vi "Cycle.vi"(8 "error in (no error)":errorcluster, 11 "BehaviorClassification In":refnum<class "BehaviorClassification.lvclass">) -> (0 "error out":errorcluster, 3 "BehaviorClassification Out":refnum<class "BehaviorClassification.lvclass">)   [LabVIEW 2010, in "BehaviorClassification.lvclass"]
uses:
  BehaviorClassification.lvclass
  BehaviorClassification.lvclass/BehaviorClassification.ctl
  MatlabExperiment/MatlabExperiment.lvclass
panel:
  in  "RewardAmount":dbl=50.0
  in  "FixationRadius":dbl=50.0
  out "Timeouts":T1={"Intertrial"=1000.0, "AcquireFixation"=1000.0, "HoldFixation"=300.0, "DelayPeriod"=1000.0, "ResponsePeriod"=1000.0}
  out "ExperimentStats":T2
  out "Cycles":dbl
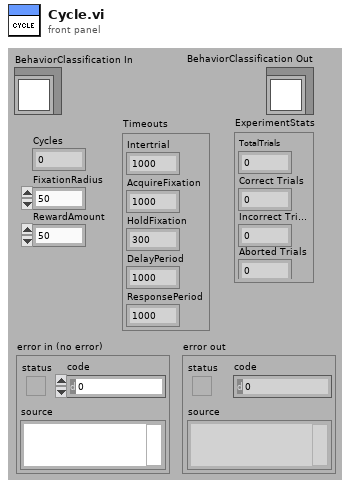
[diagram p1: front panel]
types:
  T1 = cluster{"Intertrial":dbl, "AcquireFixation":dbl, "HoldFixation":dbl, "DelayPeriod":dbl, "ResponsePeriod":dbl}
  T2 = cluster{"TotalTrials":dbl, "Correct Trials":dbl, "Incorrect Trials":dbl, "Aborted Trials":dbl}
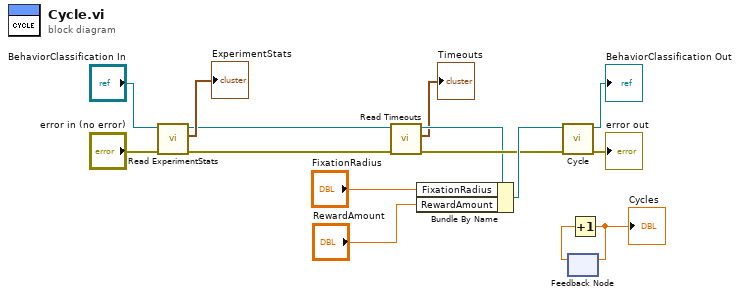
[diagram p0: block diagram]
diagram:
  n1 = call-dynamic "Read ExperimentStats.vi"("error in (no error)"="error in (no error)", "TrialBasedExperiment in"="BehaviorClassification In") -> ("error out"=w4:errorcluster, "ExperimentStats"=→"ExperimentStats":T2, "TrialBasedExperiment out"=w5:refnum<class "BehaviorClassification.lvclass">)  [unwired: 7 in]
  n2 = call-dynamic "Read Timeouts.vi"("error in (no error)"=w4, "TrialBasedExperiment in"=w5) -> ("error out"=w3:errorcluster, "Timeouts"=→"Timeouts":T1, "TrialBasedExperiment out"=w2:refnum<class "BehaviorClassification.lvclass">)  [unwired: 7 in]
  n3 = Bundle By Name(cluster=w2, "FixationRadius"="FixationRadius", "RewardAmount"="RewardAmount") -> (w8:refnum<class "BehaviorClassification.lvclass">)
  n4 = call-parent "Cycle.vi"("error in (no error)"=w3, "TrialBasedExperiment In"=w8) -> ("error out"=→"error out":errorcluster, "TrialBasedExperiment Out"=→"BehaviorClassification Out":refnum<class "BehaviorClassification.lvclass">)  [unwired: 8 in]
  n5 = feedback #1() -> (w12:dbl)  [unwired: 1 in]
  n6 = Increment(x=w12) -> (x+1=w13:dbl)
  "Cycles" <- w13
  n7 = feedback-in #1(w13) -> ()
